vi "oneMeasureAndQuit.vi"(8 "Stop":bool, 11 "Handle":u32) -> (4 "Current Incoming row":u16, 6 "SpecCount":i32)   [LabVIEW 2012]
uses:
  <vilib>/Utility/file.llb/Write To Spreadsheet File (DBL).vi
  Sciospec ISX3 Impedance Analyzer.lvlib
panel:
  out "ACK for Start CMD":u8[](array[numeric])
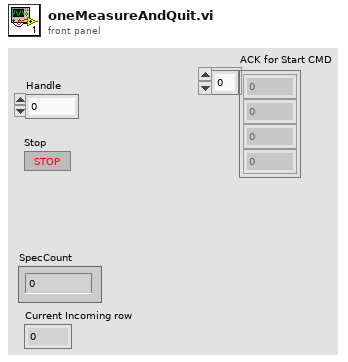
[diagram p1: front panel]
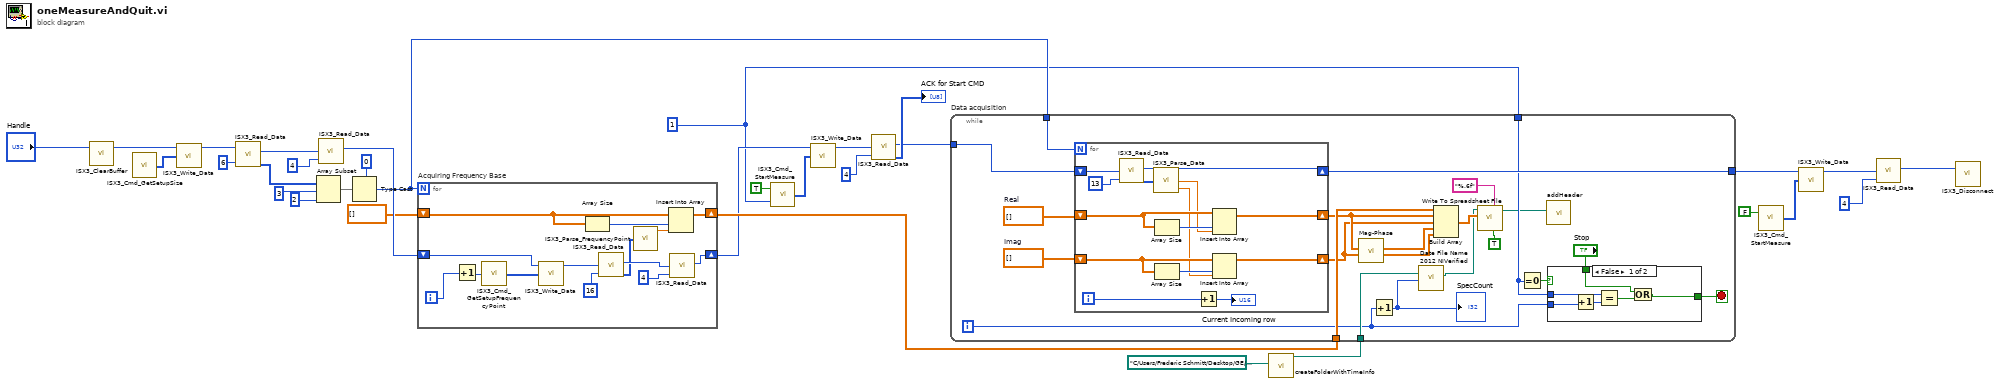
[diagram p0: block diagram]
diagram:
  w11 = u16 1 ("Number of Spectra")
  n1 = call "ISX3_ClearBuffer.vi"("Handle"="Handle") -> ("Handle"=w4:u32)  [unwired: 1 in, 1 out]
  n2 = call "ISX3_Cmd_GetSetupSize.vi"() -> ("get Setup Size Cmd"=w15:u8[])  [unwired: 1 in]
  n3 = call "ISX3_Write_Data.vi"("Data to Write"=w15, "FT_Handle"=w4) -> ("FT_Handle"=w16:u32)  [unwired: 2 in, 1 out]
  n4 = call "ISX3_Read_Data.vi"("FT_Handle"=w16, "Bytes To Read"=6) -> ("Handle"=w27:u32, "Read Data"=w25:u8[])  [unwired: 2 in, 1 out]
  n5 = Array Subset(array=w25, index=3, length=2) -> (w26:u8[])
  n6 = call "ISX3_Read_Data.vi"("FT_Handle"=w27, "Bytes To Read"=4) -> ("Handle"=w21:u32)  [unwired: 2 in, 2 out]
  n7 = Type Cast(type=u16 0, x=w26) -> (*(type *) &x=w18:u16)
  n8 = for "Acquiring Frequency Base" {
    N: w18 -> [_]
    shift-right: [w42] -> w20
    shift-left: dbl[] [] -> [w43]
    shift-right: [w39] -> w14
    shift-left: w21 -> [w37]
    i -> [w46]
    n9 = Increment(x=w46) -> (x+1=w38:i32)
    n10 = call "ISX3_Cmd_GetSetupFrequencyPoint.vi"("Row"=w38) -> ("get Setup Frequency Point Cmd"=w36:u8[])
    n11 = call "ISX3_Write_Data.vi"("Data to Write"=w36, "FT_Handle"=w37) -> ("FT_Handle"=w35:u32)  [unwired: 2 in, 1 out]
    n12 = Array Size(array=w43) -> (size(s)=w44:i32)
    n13 = call "ISX3_Read_Data.vi"("FT_Handle"=w35, "Bytes To Read"=16) -> ("Handle"=w41:u32, "Read Data"=w34:u8[])  [unwired: 2 in, 1 out]
    n14 = call "ISX3_Parse_FrequencyPoint.vi"("Array"=w34) -> ("Frequency [Hz]"=w33:sgl)  [unwired: 2 out]
    n15 = Insert Into Array(array=w43, index=w44, new element=w33) -> (w42:dbl[])
    n16 = call "ISX3_Read_Data.vi"("FT_Handle"=w41, "Bytes To Read"=4) -> ("Handle"=w39:u32)  [unwired: 2 in, 2 out]
  }
  n17 = call "ISX3_Cmd_StartMeasure.vi"("Number of Spectra"=w11, "Start/Stop"=TRUE) -> ("Start/Stop measurement cmd"=w10:u8[])
  n18 = call "ISX3_Write_Data.vi"("Data to Write"=w10, "FT_Handle"=w14) -> ("FT_Handle"=w13:u32)  [unwired: 2 in, 1 out]
  n19 = call "ISX3_Read_Data.vi"("FT_Handle"=w13, "Bytes To Read"=4) -> ("Handle"=w30:u32, "Read Data"=→"ACK for Start CMD":u8[])  [unwired: 2 in, 1 out]
  n20 = call "createFolderWithTimeInfo.vi"("Folder to save file to"=path "C:/Users/Frederic Schmitt/Desktop/GE/Sciospec Bioimpedance - Sinan/Sciospec ISX3v2/Data from LabVIEW") -> ("created path"=w3:path)  [unwired: 10 in]
  n21 = while "Data acquisition" {
    tunnel: w30 -> [w68]
    tunnel: [w65] -> w7
    tunnel: w20 -> [w59]
    tunnel: w11 -> [w63]
    tunnel: w18 -> [w60]
    tunnel: w3 -> [w55]
    i -> [w48]
    stop <- w62 stop-if-true
    w66 = dbl[] []  # Imag
    w67 = dbl[] []  # Real
    n22 = for {
      N: w60 -> [_]
      shift-right: [w88] -> w65
      shift-left: w68 -> [w89]
      shift-right: [w83] -> w53
      shift-left: w67 -> [w81]
      shift-right: [w85] -> w52
      shift-left: w66 -> [w86]
      i -> [w80]
      n23 = call "ISX3_Read_Data.vi"("FT_Handle"=w89, "Bytes To Read"=13) -> ("Handle"=w88:u32, "Read Data"=w76:u8[])  [unwired: 2 in, 1 out]
      n24 = call "ISX3_Parse_Data.vi"("Array"=w76) -> ("Real"=w78:sgl, "Imag"=w77:sgl)  [unwired: 1 out]
      n25 = Array Size(array=w81) -> (size(s)=w84:i32)
      n26 = Array Size(array=w86) -> (size(s)=w87:i32)
      n27 = Increment(x=w80) -> (x+1=→"Current Incoming row":i32)
      n28 = Insert Into Array(array=w81, index=w84, new element=w78) -> (w83:dbl[])
      n29 = Insert Into Array(array=w86, index=w87, new element=w77) -> (w85:dbl[])
    }
    n30 = call "Mag-Phase.vi"("Imag"=w52, "Re"=w53) -> ("phase"=w50:dbl[], "mag"=w51:dbl[])  [unwired: 7 in]
    n31 = Increment(x=w48) -> (x+1=w47:i32)
    "SpecCount" <- w47
    n32 = call "Date File Name 2012 NIVerified.vi"("Data Count"=w47, "Folder to save file to"=w55) -> ("New file path"=w56:path)  [unwired: 9 in]
    n33 = Build Array(w59, w53, w52, w51, w50) -> (w58:dbl[][])
    n34 = call-poly <vilib>:"Write To Spreadsheet File.vi"("transpose? (no:F)"=TRUE, "format (%.3f)"="%.6f", "2D data"=w58, "file path (dialog if empty)"=w56) -> ("new file path (Not A Path if cancelled)"=w54:path)  [unwired: 4 in]
    n35 = Equal To 0?(x=w63) -> (x = 0?=w64:bool)
    n36 = call "addHeader.vi"("file path (dialog if empty)"=w54) -> ()  [unwired: 11 in]
    n37 = case shown="False" w64 {
      tunnel: w63 -> [w74 _]
      tunnel: w48 -> [w73 _]
      tunnel: [w71 w75] -> w62
      tunnel: "Stop" -> [w70 w75]
      frame False {
        n38 = Increment(x=w73) -> (x+1=w72:i32)
        n39 = Equal?(x=w74, y=w72) -> (x = y?=w69:bool)
        n40 = Or(x=w70, y=w69) -> (x .or. y?=w71:bool)
      }
      frame True {
      }
    }
  }
  n41 = call "ISX3_Cmd_StartMeasure.vi"("Start/Stop"=FALSE) -> ("Start/Stop measurement cmd"=w8:u8[])  [unwired: 1 in]
  n42 = call "ISX3_Write_Data.vi"("Data to Write"=w8, "FT_Handle"=w7) -> ("FT_Handle"=w6:u32)  [unwired: 2 in, 1 out]
  n43 = call "ISX3_Read_Data.vi"("FT_Handle"=w6, "Bytes To Read"=4) -> ("Handle"=w5:u32)  [unwired: 2 in, 2 out]
  n44 = call "ISX3_Disconnect.vi"("FT_Handle"=w5) -> ()  [unwired: 2 in]
